vi "Configure Frequency Sweep.vi"(6 "Stop  Frequency  (1000 Hz)":dbl=1000.0 format="%#.6g", 7 "Start Frequency (100 Hz)":dbl=100.0 format="%#.6g", 8 "error in (no error)":errorcluster, 9 "Enable Frequency Sweep (T: Enable)":bool=TRUE, 10 "Channel (1: Channel 1)":u16(ring)=1 items=["Channel 1"=1, "Channel 2"=2], 11 "VISA resource name":refnum<visa-resource-name>) -> (0 "error out":errorcluster, 3 "VISA resource name out":refnum<visa-resource-name>)   [LabVIEW 2016, in "Tektronix AFG 1000 Series.lvlib"]
doc: "Configures and enables a frequency sweep. In the frequency sweep mode, the function generator steps from the start frequency to the stop frequency at a sweep rate."
uses:
  Tektronix AFG 1000 Series.lvlib
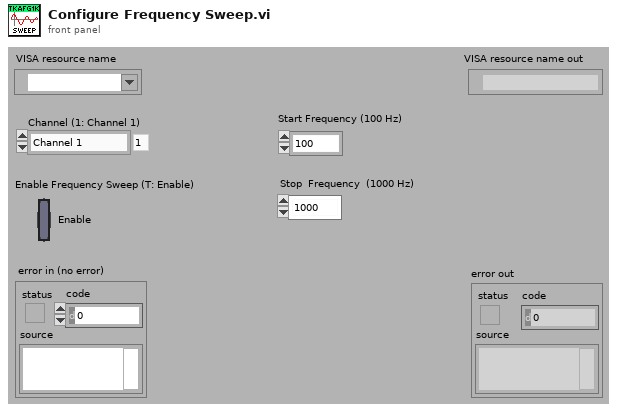
[diagram p1: front panel]
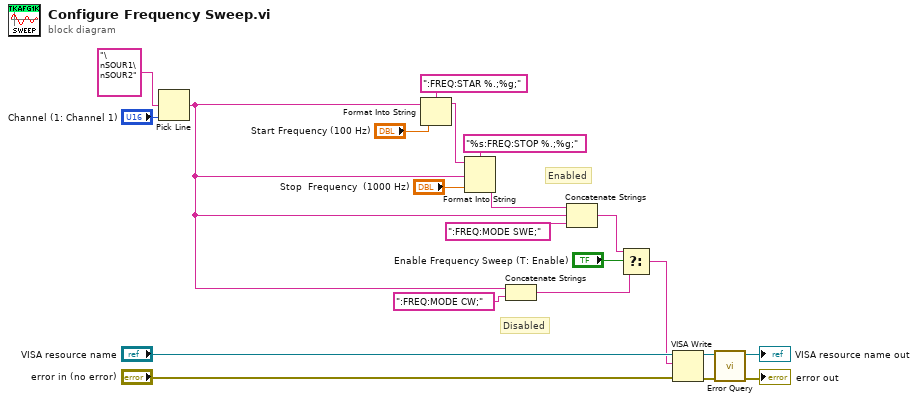
[diagram p0: block diagram]
diagram:
  # "Disabled"
  # "Enabled"
  n1 = Pick Line(multi-line string="\nSOUR1\nSOUR2" ("string (\"\")"), line index="Channel (1: Channel 1)") -> (output string=w1:string)  [unwired: 1 in]
  n2 = Format Into String(format string=":FREQ:STAR %.;%g;", initial string=w1, "Start Frequency (100 Hz)") -> (resulting string=w14:string)  [unwired: 1 in, 1 out]
  n3 = Format Into String(format string="%s:FREQ:STOP %.;%g;", initial string=w14, w1, "Stop  Frequency  (1000 Hz)") -> (resulting string=w6:string)  [unwired: 1 in, 1 out]
  n4 = Concatenate Strings(w1, ":FREQ:MODE CW;" ("Disable")) -> (w8:string)
  n5 = Concatenate Strings(w6, w1, ":FREQ:MODE SWE;" ("Enable")) -> (w10:string)
  n6 = Select(t=w10, s="Enable Frequency Sweep (T: Enable)", f=w8) -> (s? t:f=w7:string)
  n7 = VISA Write(VISA resource name="VISA resource name", write buffer=w7, error in (no error)="error in (no error)") -> (VISA resource name out=w19:refnum<visa-resource-name>, error out=w17:errorcluster)  [unwired: 1 out]
  n8 = call "Error Query.vi"("error in (no error)"=w17, "VISA resource name"=w19) -> ("error out"=→"error out":errorcluster, "VISA resource name out"=→"VISA resource name out":refnum<visa-resource-name>)  [unwired: 6 in, 2 out]
